vi "Waveform generation_dual color_plane by plane.vi"(0 "Number of Steps":dbl, 1 "488 LASER Intensity":dbl(slide) scale=0.0..10.0, 2 "SPIMA Obj Ampl":dbl, 3 "SPIMB Z- galvo amplitude":dbl, 4 "SPIMA Z-Galvo Offset":dbl(slide) scale=0.0..10.0, 5 "SPIMA Z-Galvo Amplitude":dbl(slide) scale=0.0..10.0, 6 "SPIMA Camera trigger":dbl, 7 "SPIMA Obejective Offset":dbl(slide) scale=0.0..10.0, 8 "SPIMB Obejective Offset":dbl(slide) scale=0.0..10.0, 9 "SPIMA Y-Galvo Offset":dbl(slide) scale=0.0..10.0, 10 "SPIMB Camera Trigger":dbl, 11 "561 Laser Amplitude":dbl, 14 "SPIMB Objective Amplitude":dbl(slide) scale=0.0..10.0, 15 "SPIMA Y-Galvo Amplitude":dbl(slide) scale=0.0..10.0, 21 "SPIMB Z-offset":dbl, 24 "SPIMB Y Offset":dbl, 25 "SPIMB Y Amplitude":dbl) -> (20 "DAQ 2":waveform(dbl)[](array[waveform]), 27 "DAQ1":waveform(dbl)[](array[waveform]))   [LabVIEW 2016]
uses:
  <vilib>/measure/NI_MABase.lvlib
panel:
  out "Numeric":i32
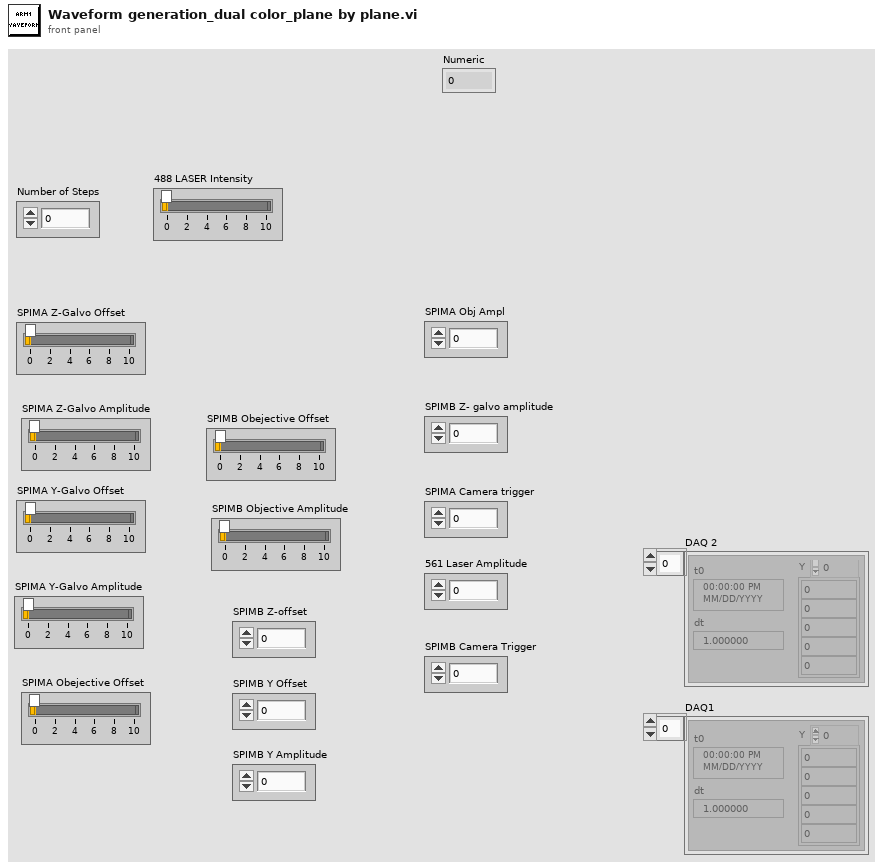
[diagram p1: front panel]
types:
  T1 = enum16{"Sine Wave", "Triangle Wave", "Square Wave", "Sawtooth Wave"}
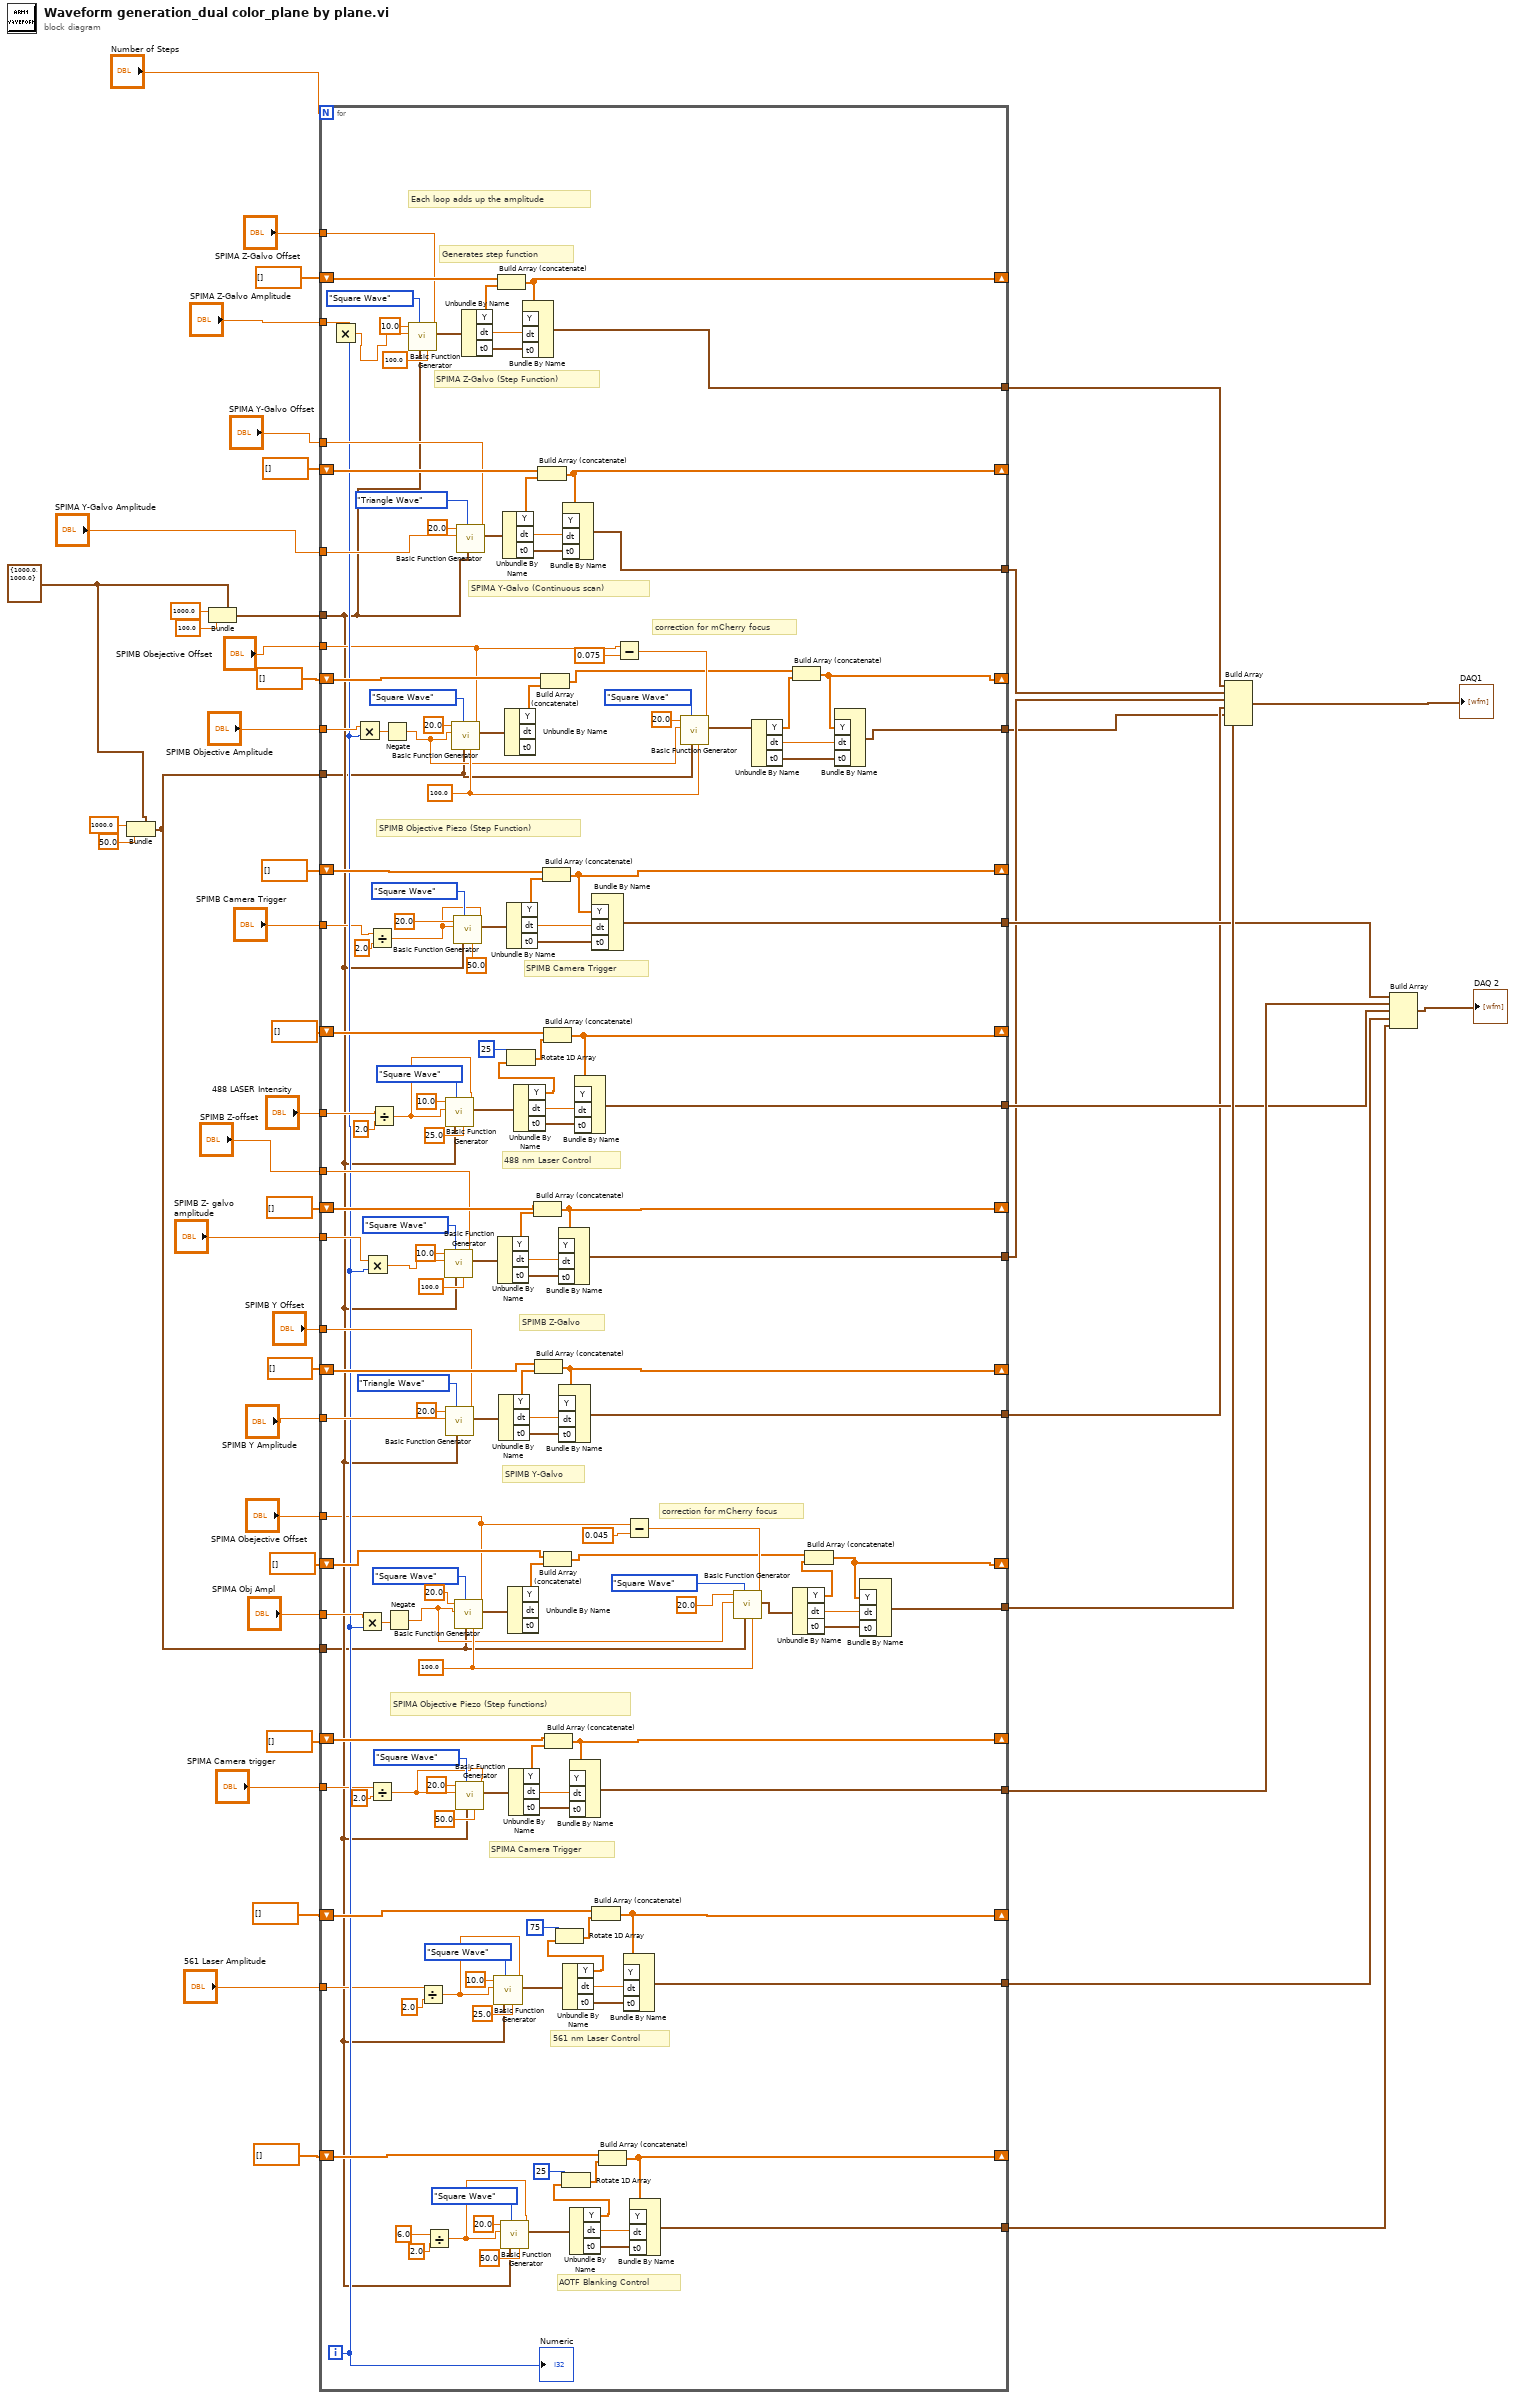
[diagram p0: block diagram]
diagram:
  w4 = cluster{"Fs":dbl, "#s":dbl} {"Fs"=1000.0, "#s"=1000.0} ("sampling info")
  n1 = Bundle(cluster=w4, "Fs"=1000.0, "#s"=50.0) -> (w1:cluster{"Fs":dbl, "#s":dbl})
  n2 = Bundle(cluster=w4, "Fs"=1000.0, "#s"=100.0) -> (w46:cluster{"Fs":dbl, "#s":dbl})
  n3 = for {
    N: "Number of Steps" -> [_]
    shift-right: [w205] -> _
    shift-left: dbl[] [] ("appended array") -> [w206]
    tunnel: [w204] -> w38
    shift-right: [w198] -> _
    shift-left: dbl[] [] ("appended array") -> [w199]
    tunnel: [w197] -> w29
    tunnel: w46 -> [w66]
    shift-right: [w51] -> _
    shift-left: dbl[] [] ("appended array") -> [w176]
    tunnel: [w69] -> w20
    shift-right: [w174] -> _
    shift-left: dbl[] [] ("appended array") -> [w175]
    tunnel: [w173] -> w28
    tunnel: "SPIMA Z-Galvo Offset" -> [w172]
    tunnel: "SPIMA Y-Galvo Offset" -> [w171]
    tunnel: "SPIMB Obejective Offset" -> [w78]
    tunnel: "488 LASER Intensity" -> [w130]
    tunnel: [w153] -> w22
    tunnel: [w152] -> w21
    tunnel: [w53] -> w37
    tunnel: [w151] -> w36
    shift-right: [w149] -> _
    shift-left: dbl[] [] ("appended array") -> [w150]
    shift-right: [w147] -> _
    shift-left: dbl[] [] ("appended array") -> [w148]
    shift-right: [w52] -> _
    shift-left: dbl[] [] ("appended array") -> [w146]
    shift-right: [w144] -> _
    shift-left: dbl[] [] ("appended array") -> [w145]
    tunnel: "SPIMA Z-Galvo Amplitude" -> [w143]
    tunnel: "SPIMB Objective Amplitude" -> [w141]
    tunnel: "SPIMA Y-Galvo Amplitude" -> [w140]
    tunnel: "SPIMA Obejective Offset" -> [w61]
    shift-right: [w134] -> _
    shift-left: dbl[] [] ("appended array") -> [w137]
    tunnel: [w138] -> w24
    tunnel: "SPIMB Z-offset" -> [w127]
    tunnel: "SPIMB Y Offset" -> [w126]
    tunnel: "SPIMB Y Amplitude" -> [w125]
    shift-right: [w98] -> _
    shift-left: dbl[] [] ("appended array") -> [w99]
    shift-right: [w96] -> _
    shift-left: dbl[] [] ("appended array") -> [w97]
    tunnel: [w95] -> w13
    tunnel: [w94] -> w12
    tunnel: "SPIMB Z- galvo amplitude" -> [w93]
    tunnel: "SPIMA Obj Ampl" -> [w92]
    tunnel: "SPIMA Camera trigger" -> [w89]
    tunnel: "561 Laser Amplitude" -> [w86]
    tunnel: "SPIMB Camera Trigger" -> [w85]
    tunnel: w1 -> [w50]
    tunnel: w1 -> [w49]
    i -> [w91]
    w65 = 100.0 ("square wave duty cycle (%)")
    w74 = 100.0 ("square wave duty cycle (%)")
    # "correction for mCherry focus"
    # "correction for mCherry focus"
    # "AOTF Blanking Control"
    # "561 nm Laser Control"
    # "Each loop adds up the amplitude"
    # "Generates step function"
    # "SPIMA Camera Trigger"
    # "SPIMA Objective Piezo (Step functions)"
    # "SPIMB Y-Galvo"
    # "SPIMB Z-Galvo"
    # "488 nm Laser Control"
    # "SPIMB Camera Trigger"
    # "SPIMB Objective Piezo (Step Function)"
    # "SPIMA Y-Galvo (Continuous scan)"
    # "SPIMA Z-Galvo (Step Function)"
    n4 = Multiply(x=w143, y=w91) -> (x*y=w81:dbl)
    n5 = Multiply(x=w141, y=w91) -> (x*y=w142:dbl)
    n6 = Multiply(x=w92, y=w91) -> (x*y=w90:dbl)
    n7 = Multiply(x=w93, y=w91) -> (x*y=w80:dbl)
    n8 = Divide(x=w85, y=2.0) -> (x/y=w83:dbl)
    n9 = Divide(x=w89, y=2.0) -> (x/y=w87:dbl)
    n10 = Divide(x=w130, y=2.0) -> (x/y=w128:dbl)
    n11 = Negate(x=w142) -> (-x=w73:dbl)
    n12 = Negate(x=w90) -> (-x=w64:dbl)
    n13 = call <vilib>:"Basic Function Generator.vi"("offset"=w172, "square wave duty cycle (%)"=100.0, "sampling info"=w66, "signal type"=T1."Square Wave", "amplitude"=w81, "frequency"=10.0) -> ("signal out"=w207:waveform(dbl))  [unwired: 3 in, 2 out]
    n14 = Divide(x=w86, y=2.0) -> (x/y=w114:dbl)
    n15 = Divide(x=6.0, y=2.0) -> (x/y=w103:dbl)
    n16 = call <vilib>:"Basic Function Generator.vi"("offset"=w127, "square wave duty cycle (%)"=100.0, "sampling info"=w66, "signal type"=T1."Square Wave", "amplitude"=w80, "frequency"=10.0) -> ("signal out"=w179:waveform(dbl))  [unwired: 3 in, 2 out]
    n17 = call <vilib>:"Basic Function Generator.vi"("offset"=w128, "square wave duty cycle (%)"=25.0, "sampling info"=w66, "signal type"=T1."Square Wave", "amplitude"=w128, "frequency"=10.0) -> ("signal out"=w139:waveform(dbl))  [unwired: 3 in, 2 out]
    n18 = call <vilib>:"Basic Function Generator.vi"("offset"=w126, "sampling info"=w66, "signal type"=T1."Triangle Wave", "amplitude"=w125, "frequency"=20.0) -> ("signal out"=w167:waveform(dbl))  [unwired: 4 in, 2 out]
    n19 = call <vilib>:"Basic Function Generator.vi"("offset"=w78, "square wave duty cycle (%)"=w74, "sampling info"=w50, "signal type"=T1."Square Wave", "amplitude"=w73, "frequency"=20.0) -> ("signal out"=w191:waveform(dbl))  [unwired: 3 in, 2 out]
    n20 = call <vilib>:"Basic Function Generator.vi"("offset"=w83, "square wave duty cycle (%)"=50.0, "sampling info"=w66, "signal type"=T1."Square Wave", "amplitude"=w83, "frequency"=20.0) -> ("signal out"=w187:waveform(dbl))  [unwired: 3 in, 2 out]
    n21 = call <vilib>:"Basic Function Generator.vi"("offset"=w61, "square wave duty cycle (%)"=w65, "sampling info"=w49, "signal type"=T1."Square Wave", "amplitude"=w64, "frequency"=20.0) -> ("signal out"=w161:waveform(dbl))  [unwired: 3 in, 2 out]
    n22 = call <vilib>:"Basic Function Generator.vi"("offset"=w87, "square wave duty cycle (%)"=50.0, "sampling info"=w66, "signal type"=T1."Square Wave", "amplitude"=w87, "frequency"=20.0) -> ("signal out"=w156:waveform(dbl))  [unwired: 3 in, 2 out]
    n23 = call <vilib>:"Basic Function Generator.vi"("offset"=w171, "sampling info"=w66, "signal type"=T1."Triangle Wave", "amplitude"=w140, "frequency"=20.0) -> ("signal out"=w200:waveform(dbl))  [unwired: 4 in, 2 out]
    n24 = Unbundle By Name(w207) -> ("Y"=w208:dbl[], "dt"=w195:dbl, "t0"=w196:timestamp)
    n25 = call <vilib>:"Basic Function Generator.vi"("offset"=w114, "square wave duty cycle (%)"=25.0, "sampling info"=w66, "signal type"=T1."Square Wave", "amplitude"=w114, "frequency"=10.0) -> ("signal out"=w120:waveform(dbl))  [unwired: 3 in, 2 out]
    n26 = Build Array (concatenate)(w206, w208) -> (w205:dbl[])
    n27 = Unbundle By Name(w179) -> ("Y"=w180:dbl[], "dt"=w177:dbl, "t0"=w178:timestamp)
    n28 = Unbundle By Name(w167) -> ("Y"=w168:dbl[], "dt"=w165:dbl, "t0"=w166:timestamp)
    n29 = call <vilib>:"Basic Function Generator.vi"("offset"=w103, "square wave duty cycle (%)"=50.0, "sampling info"=w66, "signal type"=T1."Square Wave", "amplitude"=w103, "frequency"=20.0) -> ("signal out"=w109:waveform(dbl))  [unwired: 3 in, 2 out]
    n30 = Unbundle By Name(w200) -> ("Y"=w201:dbl[], "dt"=w202:dbl, "t0"=w203:timestamp)
    n31 = Unbundle By Name(w191) -> ("Y"=w192:dbl[])  [unwired: 2 out]
    n32 = Unbundle By Name(w187) -> ("Y"=w188:dbl[], "dt"=w185:dbl, "t0"=w186:timestamp)
    n33 = Unbundle By Name(w161) -> ("Y"=w162:dbl[])  [unwired: 2 out]
    n34 = Unbundle By Name(w156) -> ("Y"=w157:dbl[], "dt"=w154:dbl, "t0"=w155:timestamp)
    n35 = Unbundle By Name(w139) -> ("Y"=w122:dbl[], "dt"=w136:dbl, "t0"=w135:timestamp)
    n36 = Rotate 1D Array(1:w122, 2:25 ("n")) -> (0:w123:dbl[])
    n37 = Bundle By Name("Y"=w205, "dt"=w195, "t0"=w196) -> (w204:waveform(dbl))  [unwired: 1 in]
    n38 = Build Array (concatenate)(w150, w180) -> (w149:dbl[])
    n39 = Build Array (concatenate)(w148, w168) -> (w147:dbl[])
    n40 = Build Array (concatenate)(w199, w201) -> (w198:dbl[])
    n41 = Build Array (concatenate)(w176, w192) -> (w68:dbl[])
    n42 = Build Array (concatenate)(w175, w188) -> (w174:dbl[])
    n43 = Build Array (concatenate)(w137, w123) -> (w134:dbl[])
    n44 = Build Array (concatenate)(w146, w162) -> (w57:dbl[])
    n45 = Build Array (concatenate)(w145, w157) -> (w144:dbl[])
    n46 = Bundle By Name("Y"=w149, "dt"=w177, "t0"=w178) -> (w153:waveform(dbl))  [unwired: 1 in]
    n47 = Bundle By Name("Y"=w147, "dt"=w165, "t0"=w166) -> (w152:waveform(dbl))  [unwired: 1 in]
    n48 = Bundle By Name("Y"=w198, "dt"=w202, "t0"=w203) -> (w197:waveform(dbl))  [unwired: 1 in]
    n49 = Unbundle By Name(w120) -> ("Y"=w111:dbl[], "dt"=w119:dbl, "t0"=w118:timestamp)
    n50 = Rotate 1D Array(1:w111, 2:75 ("n")) -> (0:w112:dbl[])
    n51 = Bundle By Name("Y"=w144, "dt"=w154, "t0"=w155) -> (w151:waveform(dbl))  [unwired: 1 in]
    n52 = Unbundle By Name(w109) -> ("Y"=w100:dbl[], "dt"=w108:dbl, "t0"=w107:timestamp)
    n53 = Rotate 1D Array(1:w100, 2:25 ("n")) -> (0:w101:dbl[])
    n54 = Bundle By Name("Y"=w134, "dt"=w136, "t0"=w135) -> (w138:waveform(dbl))  [unwired: 1 in]
    n55 = Bundle By Name("Y"=w174, "dt"=w185, "t0"=w186) -> (w173:waveform(dbl))  [unwired: 1 in]
    n56 = Build Array (concatenate)(w99, w112) -> (w98:dbl[])
    n57 = Build Array (concatenate)(w97, w101) -> (w96:dbl[])
    n58 = Subtract(x=w78, y=0.075) -> (x-y=w76:dbl)
    n59 = Bundle By Name("Y"=w98, "dt"=w119, "t0"=w118) -> (w95:waveform(dbl))  [unwired: 1 in]
    n60 = Subtract(x=w61, y=0.045) -> (x-y=w59:dbl)
    n61 = Bundle By Name("Y"=w96, "dt"=w108, "t0"=w107) -> (w94:waveform(dbl))  [unwired: 1 in]
    n62 = call <vilib>:"Basic Function Generator.vi"("offset"=w76, "square wave duty cycle (%)"=w74, "sampling info"=w50, "signal type"=T1."Square Wave", "amplitude"=w73, "frequency"=20.0) -> ("signal out"=w72:waveform(dbl))  [unwired: 3 in, 2 out]
    n63 = call <vilib>:"Basic Function Generator.vi"("offset"=w59, "square wave duty cycle (%)"=w65, "sampling info"=w49, "signal type"=T1."Square Wave", "amplitude"=w64, "frequency"=20.0) -> ("signal out"=w58:waveform(dbl))  [unwired: 3 in, 2 out]
    n64 = Unbundle By Name(w72) -> ("Y"=w67:dbl[], "dt"=w70:dbl, "t0"=w71:timestamp)
    n65 = Build Array (concatenate)(w68, w67) -> (w51:dbl[])
    n66 = Unbundle By Name(w58) -> ("Y"=w56:dbl[], "dt"=w55:dbl, "t0"=w54:timestamp)
    n67 = Build Array (concatenate)(w57, w56) -> (w52:dbl[])
    n68 = Bundle By Name("Y"=w51, "dt"=w70, "t0"=w71) -> (w69:waveform(dbl))  [unwired: 1 in]
    n69 = Bundle By Name("Y"=w52, "dt"=w55, "t0"=w54) -> (w53:waveform(dbl))  [unwired: 1 in]
    "Numeric" <- w91
  }
  n70 = Build Array(w38, w29, w22, w21, w20, w37) -> (→"DAQ1":waveform(dbl)[])
  n71 = Build Array(w28, w36, w24, w13, w12) -> (→"DAQ 2":waveform(dbl)[])
